vi "Test Save PNG (Memory).vi"(8 "error in (no error)":errorcluster) -> (0 "error out":errorcluster, 3 "Pass?":bool)   [LabVIEW 2020]
uses:
  <vilib>/picture/picture.llb/imagedata.ctl
  G-Image/G-Image.lvlib
  G-Image/Image IO/Polymorphic VIs/Load Image (Memory).vi
  G-Image/Image IO/Polymorphic VIs/Save PNG Image (Memory).vi
panel:
  out "Array":cluster{string, "new picture":picture}[](array[cluster])
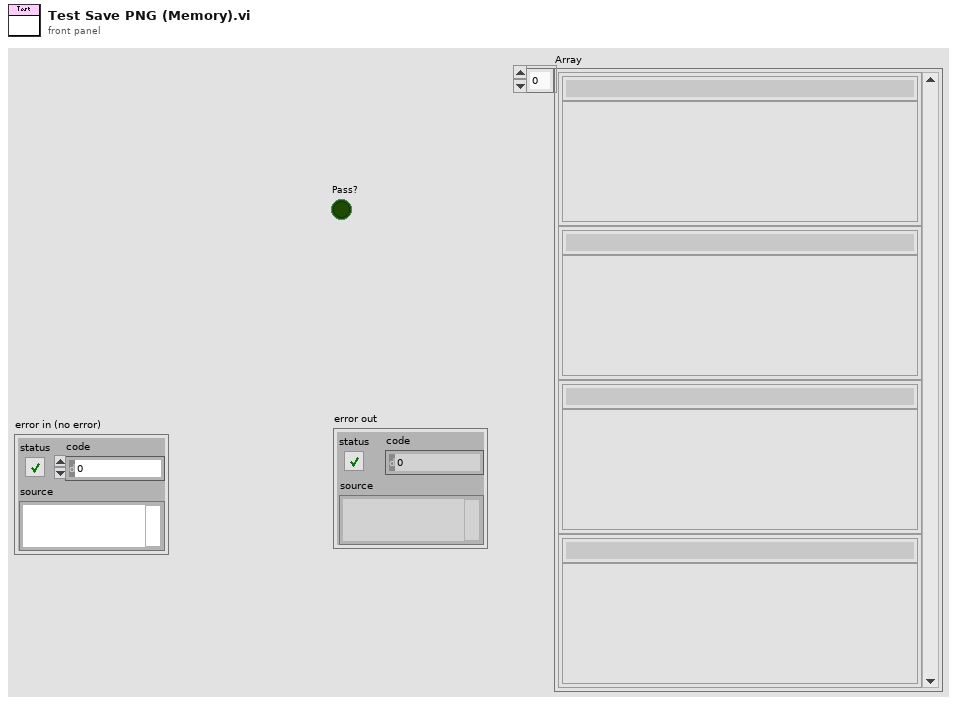
[diagram p1: front panel]
types:
  T1 = typedef "imagedata.ctl" = cluster{"image type":i32, "image depth":i32, "image":u8[], "mask":u8[], "colors":u32[], "Rectangle":cluster{"left":i16, "top":i16, "right":i16, "bottom":i16}}
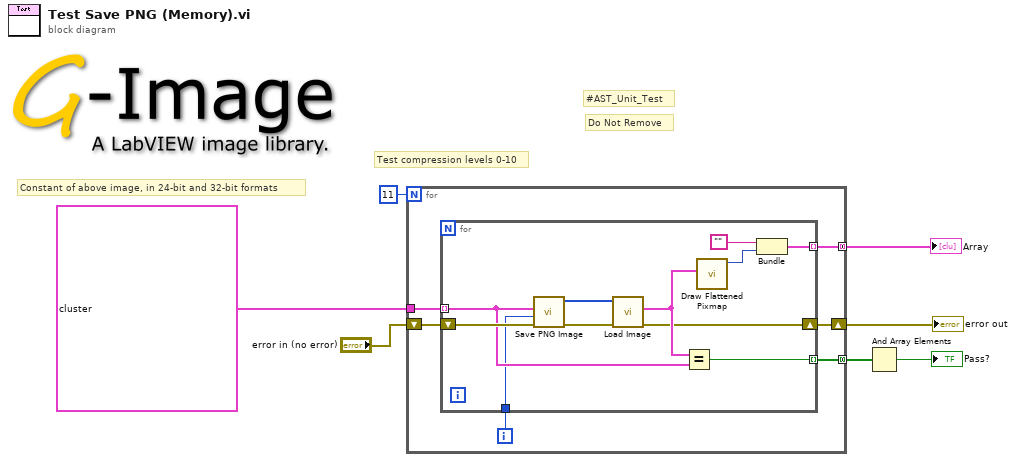
[diagram p0: block diagram]
diagram:
  # "Test compression levels 0-10"
  # "Constant of above image, in 24-bit and 32-bit formats"
  # "Do Not Remove"
  # "#AST_Unit_Test"
  n1 = for {
    N: 11 -> [_]
    tunnel: [w12] -> w6 mode=concatenating
    tunnel: [w10] -> w4 mode=concatenating
    tunnel: T1[] [{"image type"=0, "image depth"=24, "image"=array[115500 elements], "mask"=[], "colors"=[], "Rectangle"={"left"=0, "top"=0, "right"=350, "bottom"=110}}, {"image type"=0, "image depth"=32, "image"=array[154000 elements], "mask"=array[4840 elements], "colors"=[], "Rectangle"={"left"=0, "top"=0, "right"=350, "bottom"=110}}] ("Array 2") -> [w9]
    shift-right: [w11] -> w5
    shift-left: "error in (no error)" -> [w13]
    i -> [w8]
    n2 = for {
      tunnel: w9 -> [w21] mode=indexing
      shift-right: [w14] -> w11
      shift-left: w13 -> [w24]
      tunnel: [w20] -> w10 mode=indexing
      tunnel: [w17] -> w12 mode=indexing
      tunnel: w8 -> [w16]
      n3 = call-poly "Save PNG Image.vi"("error in (no error)"=w24, "Compression (6)"=w16, "Image"=w21) -> ("error out"=w22:errorcluster, "Encoded Image"=w23:u8[])  [unwired: 7 in]
      n4 = call-poly "Load Image.vi"("error in (no error)"=w22, "Encoded Image"=w23) -> ("error out"=w14:errorcluster, "Image"=w19:T1)  [unwired: 8 in]
      n5 = Equal?(x=w19, y=w21) -> (x = y?=w20:bool)
      n6 = call <vilib>:"Draw Flattened Pixmap.vi"("image data"=w19) -> ("new picture"=w18:picture)  [unwired: 8 in]
      n7 = Bundle("", "new picture"=w18) -> (w17:cluster{string, "new picture":picture})  [unwired: 1 in]
    }
  }
  "error out" <- w5
  "Array" <- w6
  n8 = And Array Elements(Boolean array=w4) -> (logical AND=→"Pass?":bool)
